vi "Word_Set_Chart_Gridelines.vi"(0 "Axes in":refnum<k7>, 1 "gridlines":T1, 5 "Type":i32(ring)=1 items=["xlCategory"=1, "xlSeriesAxis"=3, "xlValue"=2], 11 "error in":errorcluster) -> (4 "Axes out":refnum<k7>, 15 "error out":errorcluster)   [LabVIEW 2017, in "NI_ReportGenerationToolkit.lvlib"]
uses:
  <vilib>/addons/_office/NI_ReportGenerationToolkit.lvlib
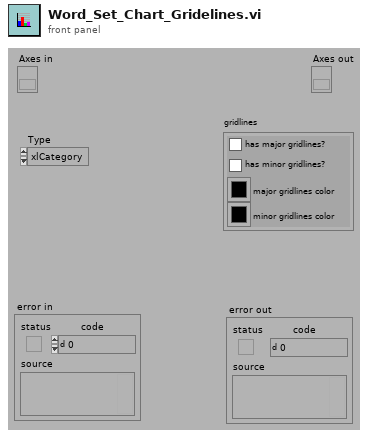
[diagram p1: front panel]
types:
  T1 = cluster{"has major gridlines?":bool, "has minor gridlines?":bool, "major gridlines color":u32, "minor gridlines color":u32}
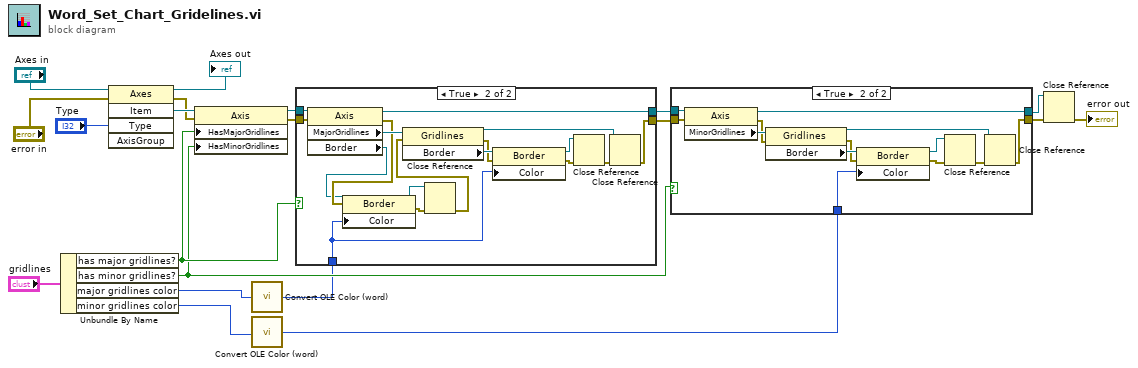
[diagram p0: block diagram]
diagram:
  n1 = Unbundle By Name("gridlines") -> ("has major gridlines?"=w5:bool, "has minor gridlines?"=w4:bool, "major gridlines color"=w3:u32, "minor gridlines color"=w2:u32)
  n2 = invoke class="Axes" method="Item"(reference="Axes in", error in="error in", "Type"="Type") -> (reference out=→"Axes out":refnum<k7>, error out=w15:errorcluster, "Item"=w17:refnum<k7>)  [unwired: 2 in, 2 out]
  n3 = property class="Axis"(reference=w17, error in=w15, "HasMajorGridlines"=w5, "HasMinorGridlines"=w4) -> (reference out=w16:refnum<k7>, error out=w14:errorcluster)
  n4 = call <vilib>:"Convert OLE Color (word).vi"("color in"=w3) -> ("color out"=w1:u32)
  n5 = call <vilib>:"Convert OLE Color (word).vi"("color in"=w2) -> ("color out"=w11:u32)
  n6 = case shown="True" w5 {
    tunnel: w16 -> [w22 w39]
    tunnel: [w22 w32] -> w13
    tunnel: [w21 w31] -> w12
    tunnel: w14 -> [w21 w30]
    tunnel: w1 -> [_ w23]
    frame False {
    }
    frame True {
      n7 = property class="Axis"(reference=w39, error in=w30) -> (reference out=w32:refnum<k7>, error out=w28:errorcluster, "MajorGridlines"=w37:refnum<k7>, "Border"=w27:refnum<k7>)
      n8 = property class="Border"(reference=w27, error in=w28, "Color"=w23) -> (reference out=w25:refnum<k7>, error out=w26:errorcluster)
      n9 = Close Reference(reference=w25, error in (no error)=w26) -> (error out=w24:errorcluster)
      n10 = property class="Gridlines"(reference=w37, error in=w24) -> (reference out=w33:refnum<k7>, error out=w29:errorcluster, "Border"=w38:refnum<k7>)
      n11 = property class="Border"(reference=w38, error in=w29, "Color"=w23) -> (reference out=w35:refnum<k7>, error out=w36:errorcluster)
      n12 = Close Reference(reference=w35, error in (no error)=w36) -> (error out=w34:errorcluster)
      n13 = Close Reference(reference=w33, error in (no error)=w34) -> (error out=w31:errorcluster)
    }
  }
  n14 = case shown="True" w4 {
    tunnel: w13 -> [w41 w54]
    tunnel: [w41 w47] -> w8
    tunnel: [w40 w46] -> w9
    tunnel: w12 -> [w40 w45]
    tunnel: w11 -> [_ w42]
    frame False {
    }
    frame True {
      n15 = property class="Axis"(reference=w54, error in=w45) -> (reference out=w47:refnum<k7>, error out=w44:errorcluster, "MinorGridlines"=w52:refnum<k7>)
      n16 = property class="Gridlines"(reference=w52, error in=w44) -> (reference out=w48:refnum<k7>, error out=w43:errorcluster, "Border"=w53:refnum<k7>)
      n17 = property class="Border"(reference=w53, error in=w43, "Color"=w42) -> (reference out=w50:refnum<k7>, error out=w51:errorcluster)
      n18 = Close Reference(reference=w50, error in (no error)=w51) -> (error out=w49:errorcluster)
      n19 = Close Reference(reference=w48, error in (no error)=w49) -> (error out=w46:errorcluster)
    }
  }
  n20 = Close Reference(reference=w8, error in (no error)=w9) -> (error out=→"error out":errorcluster)
